vi "Chopper Motor Test.vi"(7 "Measurement Started?":bool, 8 "error in (no error)":errorcluster, 11 "Session Handle in":T1) -> (0 "error out":errorcluster, 2 "Passed?":bool, 3 "Session Handle out":T1 caption="Gas")   [LabVIEW 2015, in "PAS.lvclass"]
uses:
  PAS.lvclass
  Typedefs/Session Handle.ctl
panel:
  out "Frequency":dbl
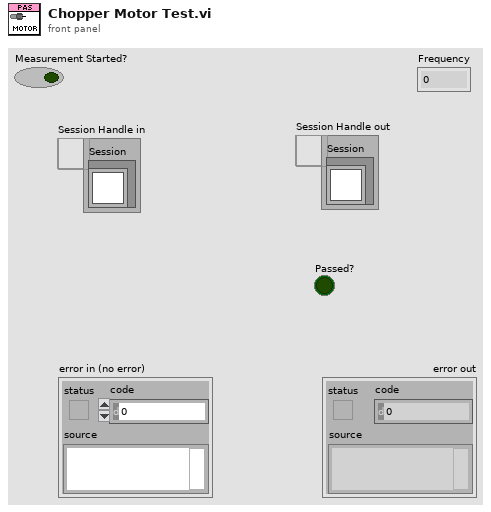
[diagram p1: front panel]
types:
  T1 = typedef "PAS.lvclass/Session Handle.ctl" = refnum<data-value>
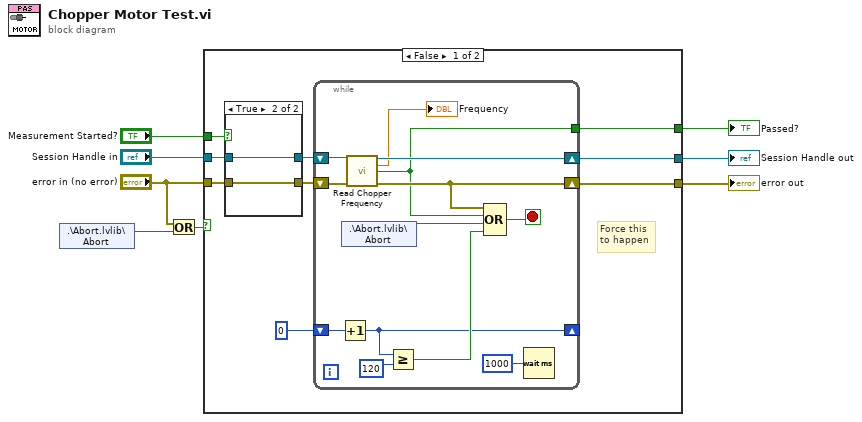
[diagram p0: block diagram]
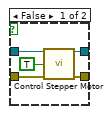
[diagram p2: hidden frame]
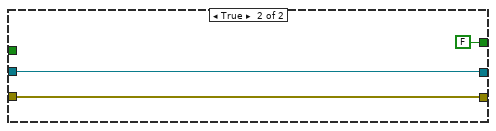
[diagram p3: hidden frame]
diagram:
  n1 = shared-variable ".\\Abort.lvlib\\Abort"() -> (w3:bool)  [unwired: 1 in, 1 out]
  n2 = Or(x="error in (no error)", y=w3) -> (x .or. y?=w2:bool)
  n3 = case shown="False" w2 {
    tunnel: [w9 w38] -> w8
    tunnel: "Session Handle in" -> [w15 w39]
    tunnel: "error in (no error)" -> [w14 w38]
    tunnel: [w13 FALSE ("Finished Ramping?")] -> w6
    tunnel: [w10 w39] -> w5
    tunnel: "Measurement Started?" -> [w11 _]
    frame False {
      # "Force this\nto happen"
      n4 = case shown="True" w11 {
        tunnel: [w22 w24] -> w17
        tunnel: [w21 w23] -> w16
        tunnel: w15 -> [w20 w24]
        tunnel: w14 -> [w19 w23]
        frame False {
          n5 = call "Control Stepper Motor.vi"("Session Handle in"=w20, "Start?"=TRUE, "error in (no error)"=w19) -> ("Session Handle out"=w22:T1, "error out"=w21:errorcluster)  [unwired: 10 in, 1 out]
        }
        frame True {
        }
      }
      n6 = while {
        shift-right: [w33] -> w9
        shift-left: w16 -> [w36]
        shift-right: [w35] -> w10
        shift-left: w17 -> [w37]
        tunnel: [w31] -> w13
        shift-right: [w27] -> _
        shift-left: u32 0 ("milliseconds to wait") -> [w30]
        stop <- w32 stop-if-true
        n7 = Increment(x=w30) -> (x+1=w27:u32)
        n8 = shared-variable ".\\Abort.lvlib\\Abort"() -> (w25:bool)  [unwired: 1 in, 1 out]
        n9 = call "Read Chopper Frequency.vi"("Session Handle in"=w37, "error in (no error)"=w36) -> ("Session Handle out"=w35:T1, "Frequency"=→"Frequency":dbl, "Finished Ramping?"=w31:bool, "error out"=w33:errorcluster)  [unwired: 9 in, 1 out]
        n10 = Greater Or Equal?(x=w27, y=u32 120) -> (x >= y?=w28:bool)
        n11 = Compound Arithmetic op=OR(w33, w31, w25, w28) -> (w32:bool)
        n12 = Wait (ms)(milliseconds to wait=u32 1000) -> ()  [unwired: 1 out]
      }
    }
    frame True {
    }
  }
  "error out" <- w8
  "Passed?" <- w6
  "Session Handle out" <- w5
